vi "Arc_mic_v1.vi"() -> ()   [LabVIEW 2014]
uses:
  <vilib>/Instr/_visa.llb/VISA Set IO Buffer Mask.ctl
  <vilib>/Instr/_visa.llb/VISA Flush IO Buffer Mask.ctl
  <vilib>/Instr/_visa.llb/VISA Configure Serial Port (Instr).vi
panel:
  out "Received_bytes":i32(graph)
  out "Real time":timestamp
  out "Virsutinis mic":i32[](graph)
  out "B mic":i32[](graph)
  out "A mic":i32[](graph)
  in  "milliseconds to wait":u32=500
  in  "stop":bool
  in  "VISA resource name":refnum<visa-resource-name>
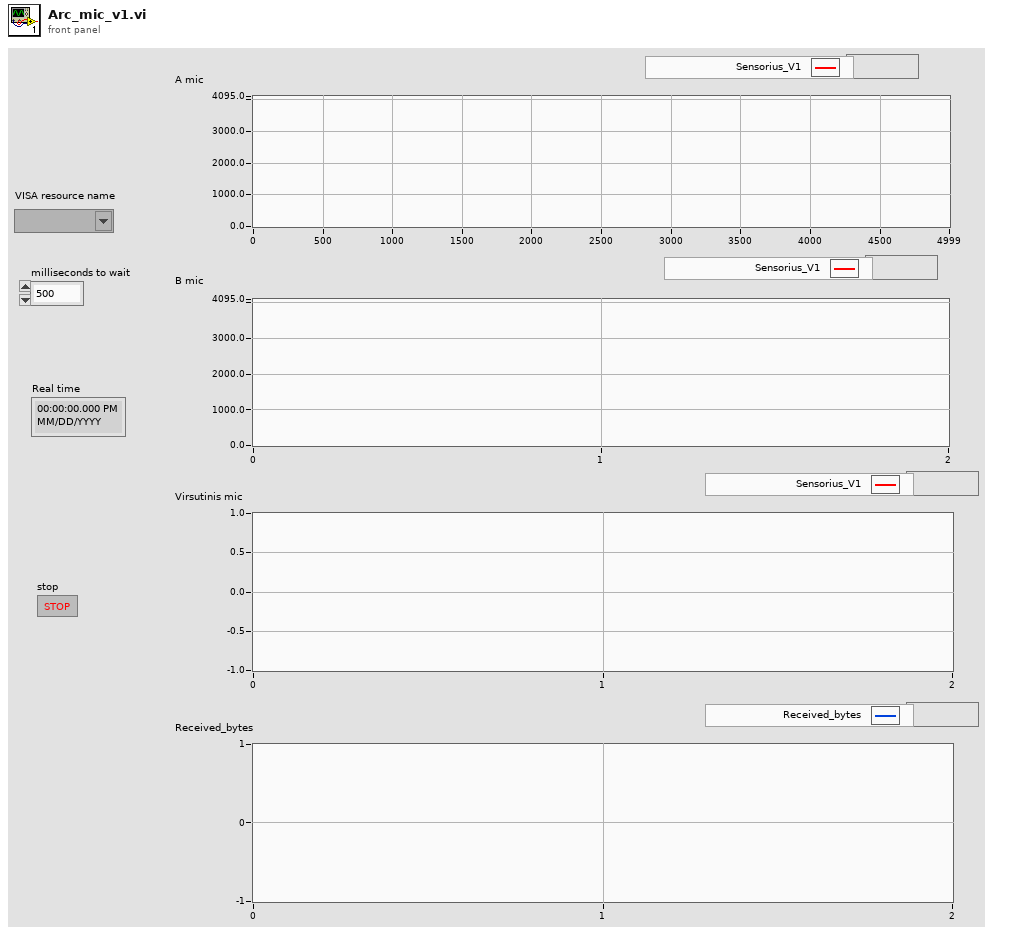
[diagram p1: front panel]
types:
  T1 = typedef "VISA Set IO Buffer Mask.ctl" = u16
  T2 = typedef "VISA Flush IO Buffer Mask.ctl" = u16
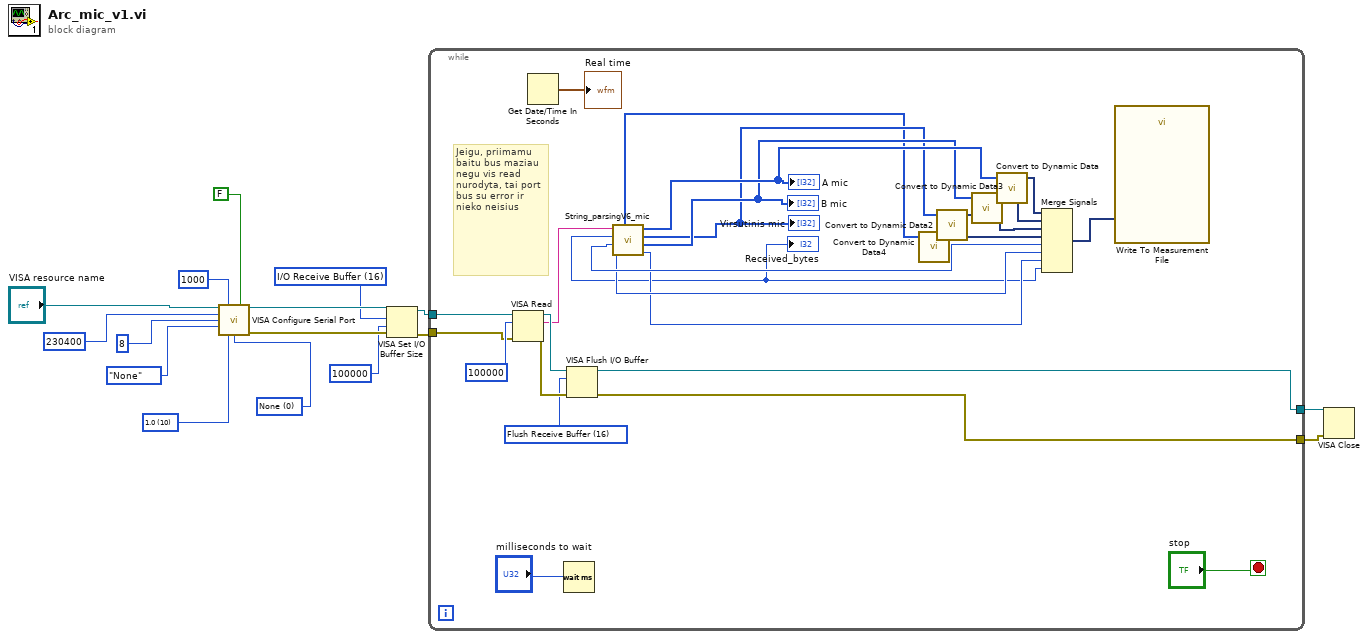
[diagram p0: block diagram]
diagram:
  w6 = T1 16 items=["I/O Receive Buffer"=16, "I/O Transmit Buffer"=32, "I/O Receive and Transmit Buffer"=48] ("Mask")
  w12 = u16 0 items=["None", "XON/XOFF", "RTS/CTS", "XON/XOFF & RTS/CTS", "DTR/DSR", "XON/XOFF & DTR/DSR"] ("flow control (0:none)")
  w13 = u16 10 items=["1.0"=10, "1.5"=15, "2.0"=20] ("stop bits (10: 1 bit)")
  n1 = call-poly "VISA Configure Serial Port"("VISA resource name"="VISA resource name", "timeout (10sec)"=u32 1000, "Enable Termination\nChar (T)"=FALSE ("Enable Termination\nChar (T)"), "baud rate (9600)"=u32 230400, "data bits (8)"=u16 8, "parity (0:none)"=enum16{"None", "Odd", "Even", "Mark", "Space"}."None", "stop bits (10: 1 bit)"=w13, "flow control (0:none)"=w12) -> ("VISA resource name out"=w8:refnum<visa-resource-name>, "error out"=w9:errorcluster)  [unwired: 6 in]
  n2 = VISA Set I/O Buffer Size(VISA resource name=w8, mask (16)=w6, size (4096)=u32 100000, error in (no error)=w9) -> (VISA resource name out=w3:refnum<visa-resource-name>, error out=w5:errorcluster)
  n3 = while {
    tunnel: w3 -> [w41]
    tunnel: w5 -> [w38]
    tunnel: [w33] -> w2
    tunnel: [w32] -> w1
    stop <- "stop" stop-if-true
    w35 = T2 16 items=["Flush Receive Buffer"=16, "Write Transmit Buffer to Device"=32, "Flush Receive Buffer (No I/O)"=64, "Flush Transmit Buffer"=128] ("Mask")
    # "Jeigu, priimamu baitu bus maziau negu vis read nurodyta, tai port bus su error ir nieko neisius"
    n4 = VISA Read(VISA resource name=w41, byte count=u32 100000, error in (no error)=w38) -> (VISA resource name out=w37:refnum<visa-resource-name>, read buffer=w26:string, error out=w36:errorcluster)  [unwired: 1 out]
    n5 = Get Date/Time In Seconds() -> (seconds since 1Jan1904=→"Real time":timestamp)
    n6 = Wait (ms)(milliseconds to wait="milliseconds to wait") -> ()  [unwired: 1 out]
    n7 = VISA Flush I/O Buffer(VISA resource name=w37, mask (16)=w35, error in (no error)=w36) -> (VISA resource name out=w33:refnum<visa-resource-name>, error out=w32:errorcluster)
    n8 = call "String_parsingV6_mic.vi"("input string"=w26) -> ("hour"=w18:i32, "V2"=w24:i32[], "V3"=w23:i32[], "V1"=w25:i32[], "timeStamp_ms"=w22:i32[], "minute"=w19:i32, "sekundes"=w20:i32, "size(s)"=w17:i32)  [unwired: 1 in]
    "A mic" <- w25
    "B mic" <- w24
    "Virsutinis mic" <- w23
    "Received_bytes" <- w17
    n9 = call "Convert to Dynamic Data4"("Array"=w22) -> ("Dynamic Data Type"=w21:dynamicdata)  [unwired: 3 in]
    n10 = call "Convert to Dynamic Data2"("Array"=w23) -> ("Dynamic Data Type"=w29:dynamicdata)  [unwired: 3 in]
    n11 = call "Convert to Dynamic Data3"("Array"=w24) -> ("Dynamic Data Type"=w28:dynamicdata)  [unwired: 3 in]
    n12 = call "Convert to Dynamic Data"("Array"=w25) -> ("Dynamic Data Type"=w31:dynamicdata)  [unwired: 3 in]
    n13 = Merge Signals(w31, w28, w29, w21, w20, w19, w18, w17) -> (w30:dynamicdata)
    n14 = call "Write To Measurement File"("Signals"=w30) -> ()  [unwired: 16 in, 3 out]
  }
  n15 = VISA Close(VISA resource name=w2, error in (no error)=w1) -> ()  [unwired: 1 out]
